vi "询问命令拆分.vi"(0 "报文":string, 10 "功能码":u8) -> (16 "拆分报告文本":T2, 18 "类别":string(combo)="16", 19 "拆分信息-数据":T1)   [LabVIEW 2019, in "MainPage.lvlib" / "MainPage.lvclass"]
uses:
  MainPage.lvclass
panel:
  # "需要前置判断CRC判定\n需要前置判断CRC判定\n需要前置判断CRC判定"
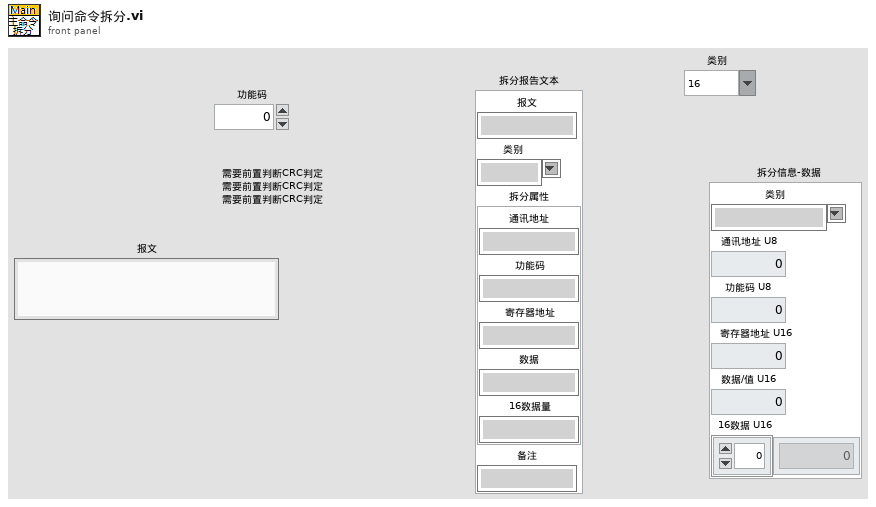
[diagram p1: front panel]
types:
  T1 = cluster{"类别":string, "通讯地址 U8":u8, "功能码 U8":u8, "寄存器地址 U16":u16, "数据/值 U16":u16, "16数据 U16":u16[]}
  T2 = cluster{"报文":string, "类别":string, "拆分属性":cluster{"通讯地址":string, "功能码":string, "寄存器地址":string, "数据":string, "16数据量":string}, "备注":string}
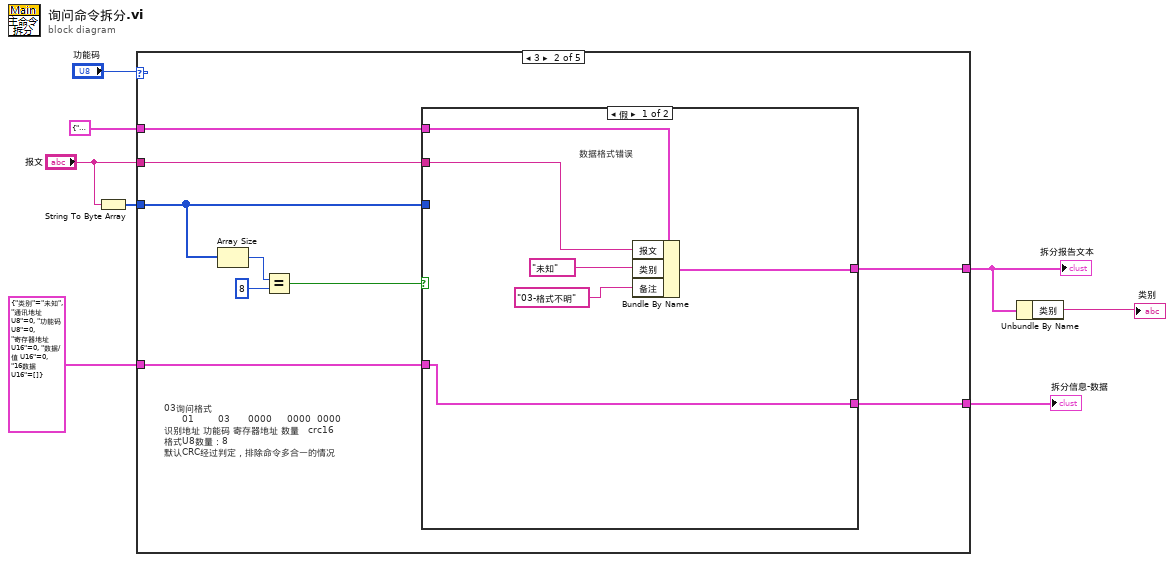
[diagram p0: block diagram]
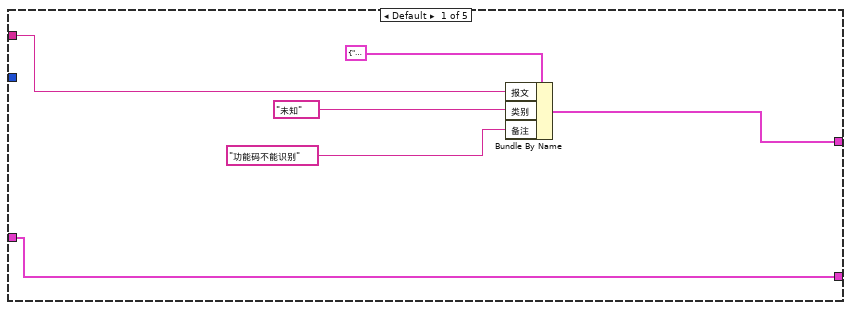
[diagram p2: hidden frame]
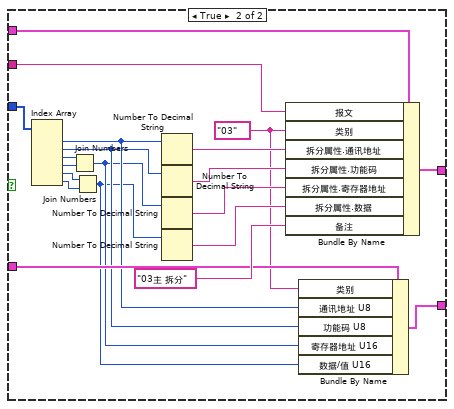
[diagram p3: hidden frame]
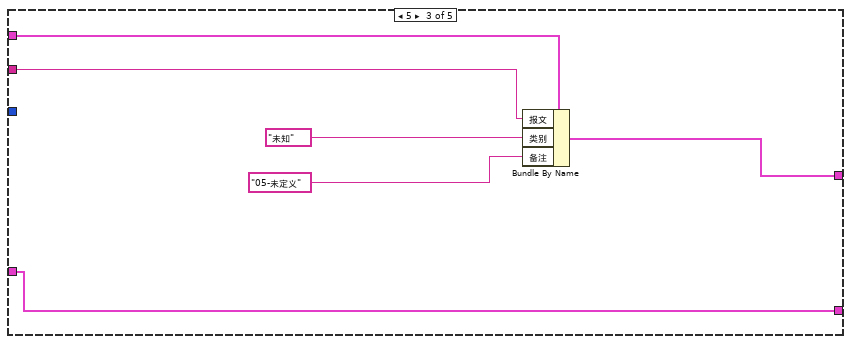
[diagram p4: hidden frame]
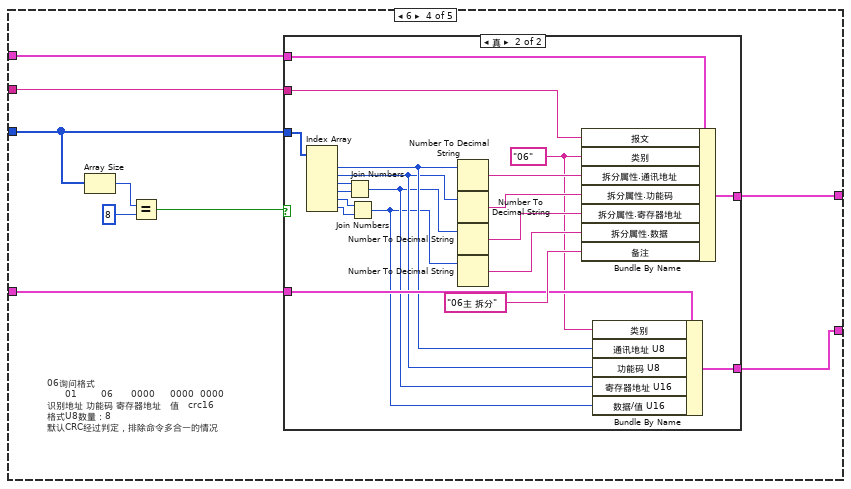
[diagram p5: hidden frame]
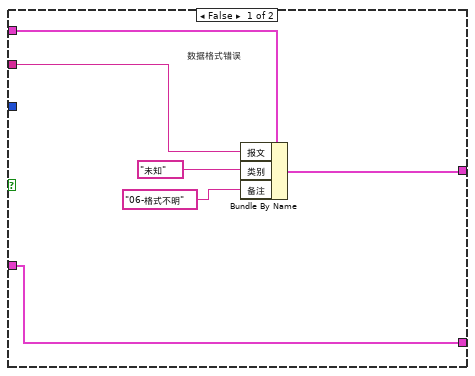
[diagram p6: hidden frame]
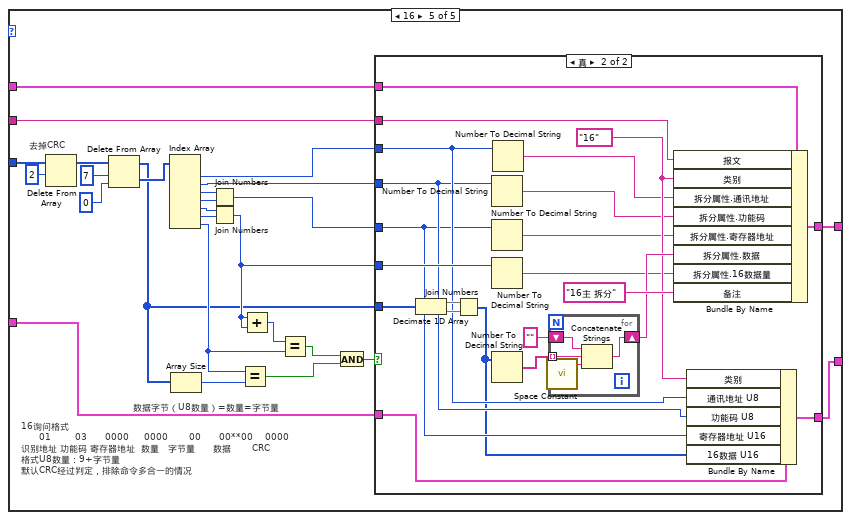
[diagram p7: hidden frame]
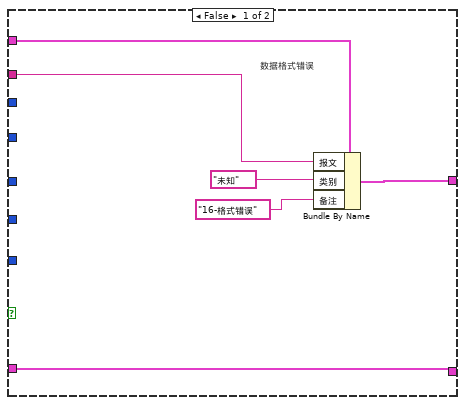
[diagram p8: hidden frame]
diagram:
  n1 = String To Byte Array(string="报文") -> (unsigned byte array=w2:u8[])
  n2 = case shown="3" "功能码" {
    tunnel: "报文" -> [w11 w20 w53 w64 w111]
    tunnel: w2 -> [_ w19 _ w59 w116]
    tunnel: [w10 w18 w55 w62 w109] -> w6
    tunnel: T2 {"报文"="", "类别"="", "拆分属性"={"通讯地址"="", "功能码"="", "寄存器地址"="", "数据"="", "16数据量"=""}, "备注"=""} ("拆分报告") -> [_ w17 w54 w63 w110]
    tunnel: T1 {"类别"="未知", "通讯地址 U8"=0, "功能码 U8"=0, "寄存器地址 U16"=0, "数据/值 U16"=0, "16数据 U16"=[]} ("拆分信息-数据") -> [w9 w16 w50 w57 w98]
    tunnel: [w9 w15 w50 w56 w93] -> w3
    frame Default {
      n3 = Bundle By Name(cluster=T2 {"报文"="", "类别"="", "拆分属性"={"通讯地址"="", "功能码"="", "寄存器地址"="", "数据"="", "16数据量"=""}, "备注"=""} ("拆分报告"), "报文"=w11, "类别"="未知", "备注"="功能码不能识别") -> (w10:T2)
    }
    frame 3 {
      # "03询问格式\n      01        03      0000     0000  0000\n识别地址 功能码 寄存器地址 数量   crc16\n格式U8数量：8\n默认CRC经过判定，排除命令多合一的情况"
      n4 = Array Size(array=w19) -> (size(s)=w23:i32)
      n5 = Equal?(x=w23, y=8) -> (x = y?=w21:bool)
      n6 = case shown="假" w21 {
        tunnel: w20 -> [w29 w48]
        tunnel: w19 -> [_ w47]
        tunnel: [w26 w49] -> w18
        tunnel: w17 -> [w25 w37]
        tunnel: w16 -> [w24 w36]
        tunnel: [w24 w35] -> w15
        frame False {
          # "数据格式错误"
          n7 = Bundle By Name(cluster=w25, "报文"=w29, "类别"="未知", "备注"="03-格式不明") -> (w26:T2)
        }
        frame True {
          w34 = "03" ("类别")
          n8 = Index Array(array=w47) -> (element #1=w33:u8, element #2=w32:u8, element #3=w44:u8, element #4=w43:u8, element #5=w41:u8, element #6=w40:u8)  [unwired: 6 in]
          n9 = Join Numbers(hi=w44, lo=w43) -> ((hi.lo)=w31:u16)
          n10 = Join Numbers(hi=w41, lo=w40) -> ((hi.lo)=w30:u16)
          n11 = Number To Decimal String(number=w33) -> (decimal integer string=w46:string)  [unwired: 1 in]
          n12 = Number To Decimal String(number=w32) -> (decimal integer string=w45:string)  [unwired: 1 in]
          n13 = Number To Decimal String(number=w31) -> (decimal integer string=w42:string)  [unwired: 1 in]
          n14 = Number To Decimal String(number=w30) -> (decimal integer string=w39:string)  [unwired: 1 in]
          n15 = Bundle By Name(cluster=w37, "报文"=w48, "类别"=w34, "拆分属性.通讯地址"=w46, "拆分属性.功能码"=w45, "拆分属性.寄存器地址"=w42, "拆分属性.数据"=w39, "备注"="03主 拆分") -> (w49:T2)
          n16 = Bundle By Name(cluster=w36, "类别"=w34, "通讯地址 U8"=w33, "功能码 U8"=w32, "寄存器地址 U16"=w31, "数据/值 U16"=w30) -> (w35:T1)
        }
      }
    }
    frame 5 {
      n17 = Bundle By Name(cluster=w54, "报文"=w53, "类别"="未知", "备注"="05-未定义") -> (w55:T2)
    }
    frame 6 {
      # "06询问格式\n      01        06      0000     0000  0000\n识别地址 功能码 寄存器地址   值   crc16\n格式U8数量：8\n默认CRC经过判定，排除命令多合一的情况"
      n18 = Array Size(array=w59) -> (size(s)=w61:i32)
      n19 = Equal?(x=w61, y=8) -> (x = y?=w58:bool)
      n20 = case shown="真" w58 {
        tunnel: w64 -> [w70 w89]
        tunnel: w59 -> [_ w88]
        tunnel: [w67 w90] -> w62
        tunnel: w63 -> [w66 w78]
        tunnel: w57 -> [w65 w77]
        tunnel: [w65 w76] -> w56
        frame False {
          # "数据格式错误"
          n21 = Bundle By Name(cluster=w66, "报文"=w70, "类别"="未知", "备注"="06-格式不明") -> (w67:T2)
        }
        frame True {
          w75 = "06" ("类别")
          n22 = Index Array(array=w88) -> (element #1=w74:u8, element #2=w73:u8, element #3=w85:u8, element #4=w84:u8, element #5=w82:u8, element #6=w81:u8)  [unwired: 6 in]
          n23 = Join Numbers(hi=w85, lo=w84) -> ((hi.lo)=w72:u16)
          n24 = Join Numbers(hi=w82, lo=w81) -> ((hi.lo)=w71:u16)
          n25 = Number To Decimal String(number=w74) -> (decimal integer string=w87:string)  [unwired: 1 in]
          n26 = Number To Decimal String(number=w73) -> (decimal integer string=w86:string)  [unwired: 1 in]
          n27 = Number To Decimal String(number=w72) -> (decimal integer string=w83:string)  [unwired: 1 in]
          n28 = Number To Decimal String(number=w71) -> (decimal integer string=w80:string)  [unwired: 1 in]
          n29 = Bundle By Name(cluster=w78, "报文"=w89, "类别"=w75, "拆分属性.通讯地址"=w87, "拆分属性.功能码"=w86, "拆分属性.寄存器地址"=w83, "拆分属性.数据"=w80, "备注"="06主 拆分") -> (w90:T2)
          n30 = Bundle By Name(cluster=w77, "类别"=w75, "通讯地址 U8"=w74, "功能码 U8"=w73, "寄存器地址 U16"=w72, "数据/值 U16"=w71) -> (w76:T1)
        }
      }
    }
    frame 16 {
      # "数据字节（U8数量）=数量=字节量"
      # "去掉CRC"
      # "16询问格式\n      01        03      0000     0000       00      00**00    0000\n识别地址 功能码 寄存器地址  数量   字节量      数据       CRC\n格式U8数量：9+字节量\n默认CRC经过判定，排除命令多合一的情况"
      n31 = Delete From Array(array=w116, length=2 ("长度")) -> (array with subset deleted=w114:u8[])  [unwired: 1 in, 1 out]
      n32 = Delete From Array(array=w114, length=7 ("长度"), index=0 ("索引")) -> (deleted portion=w92:u8[], array with subset deleted=w91:u8[])
      n33 = Index Array(array=w92) -> (element #1=w94:u8, element #2=w95:u8, element #3=w100:u8, element #4=w99:u8, element #5=w108:u8, element #6=w107:u8, element #7=w104:u8)  [unwired: 7 in]
      n34 = Array Size(array=w91) -> (size(s)=w106:i32)
      n35 = Join Numbers(hi=w100, lo=w99) -> ((hi.lo)=w96:u16)
      n36 = Join Numbers(hi=w108, lo=w107) -> ((hi.lo)=w97:u16)
      n37 = Equal?(x=w104, y=w106) -> (x = y?=w102:bool)
      n38 = Add(x=w97, y=w97) -> (x+y=w105:u16)
      n39 = Equal?(x=w105, y=w104) -> (x = y?=w103:bool)
      n40 = And(x=w103, y=w102) -> (x .and. y?=w101:bool)
      n41 = case shown="真" w101 {
        tunnel: w111 -> [w122 w143]
        tunnel: [w119 w144] -> w109
        tunnel: w110 -> [w118 w142]
        tunnel: w91 -> [_ w138]
        tunnel: w98 -> [w117 w134]
        tunnel: w97 -> [_ w132]
        tunnel: w96 -> [_ w125]
        tunnel: w95 -> [_ w126]
        tunnel: w94 -> [_ w127]
        tunnel: [w117 w123] -> w93
        frame False {
          # "数据格式错误"
          n42 = Bundle By Name(cluster=w118, "报文"=w122, "类别"="未知", "备注"="16-格式错误") -> (w119:T2)
        }
        frame True {
          w133 = "16" ("类别")
          n43 = Decimate 1D Array(w138) -> (w140:u8[], w139:u8[])
          n44 = Join Numbers(hi=w140, lo=w139) -> ((hi.lo)=w124:u16[])
          n45 = Number To Decimal String(number=w126) -> (decimal integer string=w129:string)  [unwired: 1 in]
          n46 = Number To Decimal String(number=w125) -> (decimal integer string=w130:string)  [unwired: 1 in]
          n47 = Number To Decimal String(number=w132) -> (decimal integer string=w131:string)  [unwired: 1 in]
          n48 = Number To Decimal String(number=w124) -> (decimal integer string=w137:string[])  [unwired: 1 in]
          n49 = Number To Decimal String(number=w127) -> (decimal integer string=w128:string)  [unwired: 1 in]
          n50 = for {
            tunnel: w137 -> [w148] mode=indexing
            shift-right: [w146] -> w135
            shift-left: "" -> [w147]
            n51 = call <vilib>:"Space Constant.vi"() -> ("String"=w145:string)
            n52 = Concatenate Strings(w147, w148, w145) -> (w146:string)
          }
          n53 = Bundle By Name(cluster=w142, "报文"=w143, "类别"=w133, "拆分属性.通讯地址"=w128, "拆分属性.功能码"=w129, "拆分属性.寄存器地址"=w130, "拆分属性.数据"=w135, "拆分属性.16数据量"=w131, "备注"="16主 拆分") -> (w144:T2)
          n54 = Bundle By Name(cluster=w134, "类别"=w133, "通讯地址 U8"=w127, "功能码 U8"=w126, "寄存器地址 U16"=w125, "16数据 U16"=w124) -> (w123:T1)
        }
      }
    }
  }
  "拆分报告文本" <- w6
  "拆分信息-数据" <- w3
  n55 = Unbundle By Name(w6) -> ("类别"=→"类别":string)
